vi "Patch data preview core.vi"(6 "Global cycle number among all trials":i32, 9 "Channel to load":enum16{"Red", "Green"}(ring)) -> (1 "Image ref (montage)":T1, 2 "Array":T1[](array[typedef]), 3 "Next state":T2=enum."Idle")   [LabVIEW 2020]
uses:
  Typedefs/Patch viewer internal cluster.ctl
  <vilib>/vision/Image Controls.llb/IMAQ Image.ctl
  Typedefs/Patch viewer states.ctl
  Typedefs/Read Write Enum.ctl
  User Interface/Visualisation/Timelapse Viewer/Globals/gl_Time series viewer globals.vi
  <vilib>/vision/NI_Vision_Development_Module.lvlib
panel:
  out "Array 2":T1[](array[plugin-control])
  out "Coordinates of montage positions":cluster{"X\n\nY":i32[]}[](array[cluster])
  out "Register cluster":T3
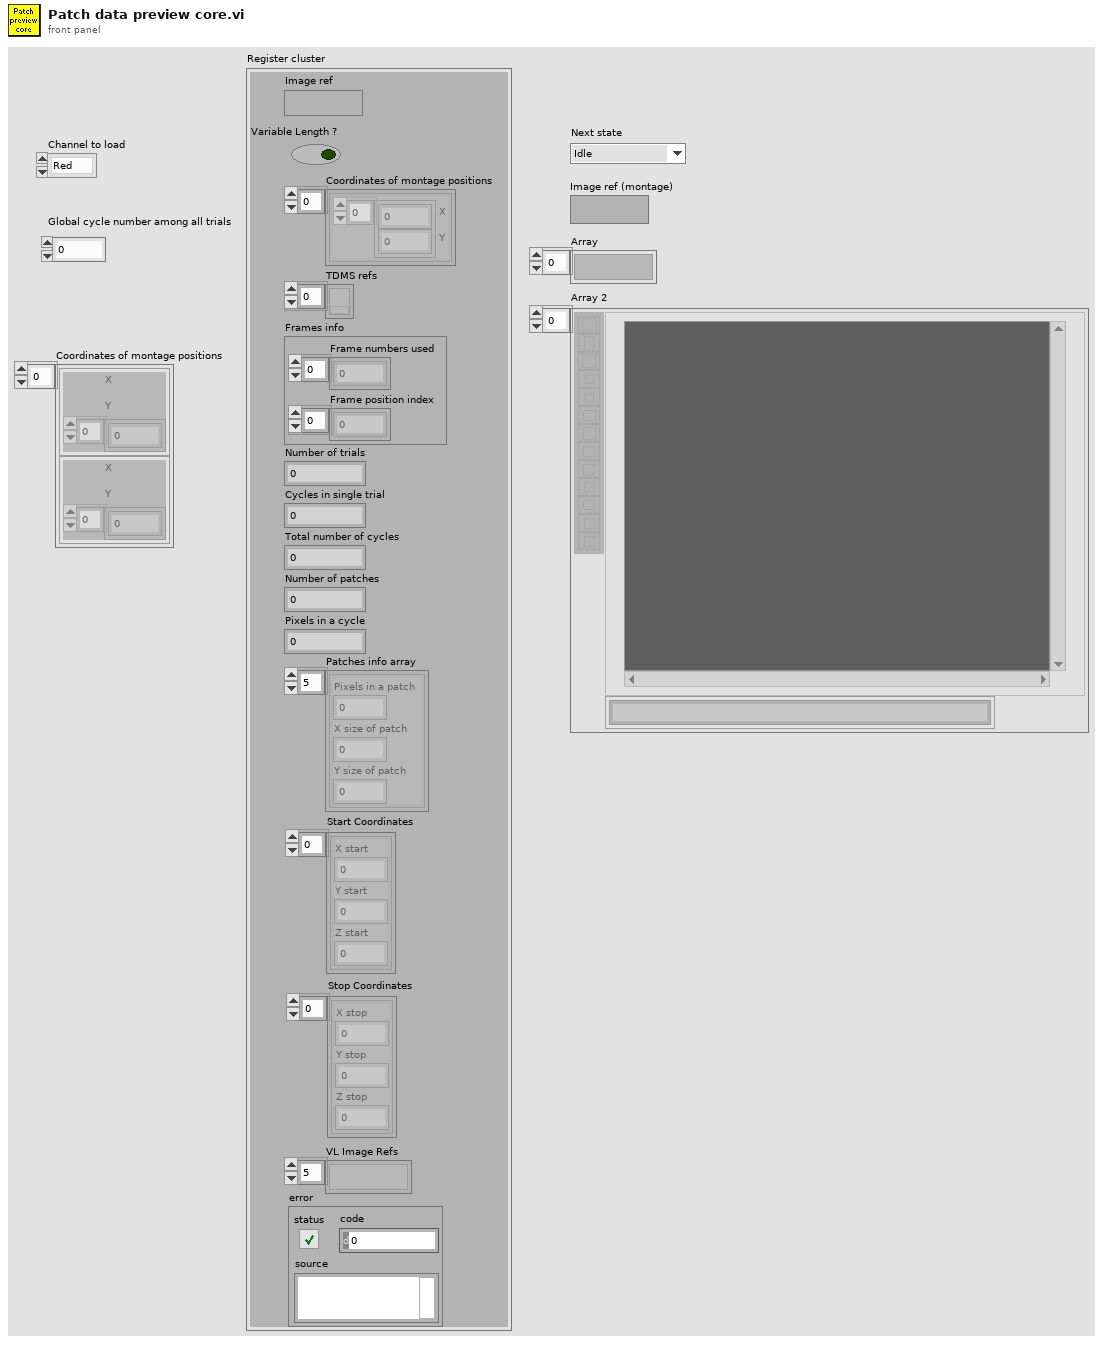
[diagram p1: front panel]
types:
  T1 = typedef "IMAQ Image.ctl" = refnum<image>
  T2 = typedef "Patch viewer states.ctl" = enum16{"Initialise", "Refresh", "Idle", "Error"}
  T3 = typedef "Patch viewer internal cluster.ctl" = cluster{"Image ref":T1, "Variable Length ?":bool, "Coordinates of montage positions":cluster{"X\n\nY":i32[]}[], "TDMS refs":refnum<k34>[], "Frames info":cluster{"Frame numbers used":i32[], "Frame position index":i32[]}, "Number of trials":i32, "Cycles in single trial":i32, "Total number of cycles":i32, "Number of patches":i32, "Pixels in a cycle":i32, "Patches info array":cluster{"Pixels in a patch":i32, "X size of patch":i32, "Y size of patch":i32}[], "Start Coordinates":cluster{"X start":i32, "Y start":i32, "Z start":i32}[], "Stop Coordinates":cluster{"X stop":i32, "Y stop":i32, "Z stop":i32}[], "VL Image Refs":T1[], "error":errorcluster}
  T4 = typedef "Read Write Enum.ctl" = enum16{"Read", "Write"}
  T5 = typedef "Image Type" = u32
  T6 = cluster{"Frame numbers used":i32[], "Frame position index":i32[]}
  T7 = cluster{"Pixels in a patch":i32, "X size of patch":i32, "Y size of patch":i32}[]
  T8 = typedef "Time series viewer refs.ctl" = cluster{"This VI":refnum<vi>, "Image control":refnum<vi>, "AVI Mode ind":refnum<vi>, "Play":refnum<vi>, "Stop":refnum<vi>, "Back":refnum<vi>, "Scrollbar":refnum<vi>, "Video length info":refnum<vi>, "Expected speed values":refnum<vi>, "Intensity":refnum<vi>, "Path":refnum<vi>, "Selection sliders":refnum<vi>, "Speed Graph ref":refnum<vi>, "Frame rate set (fps)":refnum<vi>, "Number of rows to generate":refnum<vi>, "VL Image Array":refnum<vi>, "Image Scrollbar":refnum<vi>, "Channel to load":refnum<vi>, "Colour":refnum<vi>}
  T9 = cluster{"X start":i32, "Y start":i32, "Z start":i32}[]
  T10 = cluster{"X stop":i32, "Y stop":i32, "Z stop":i32}[]
  T11 = typedef "Channel to load.ctl" = enum16{"Show red channel", "Show green channel", "Show both channels"}
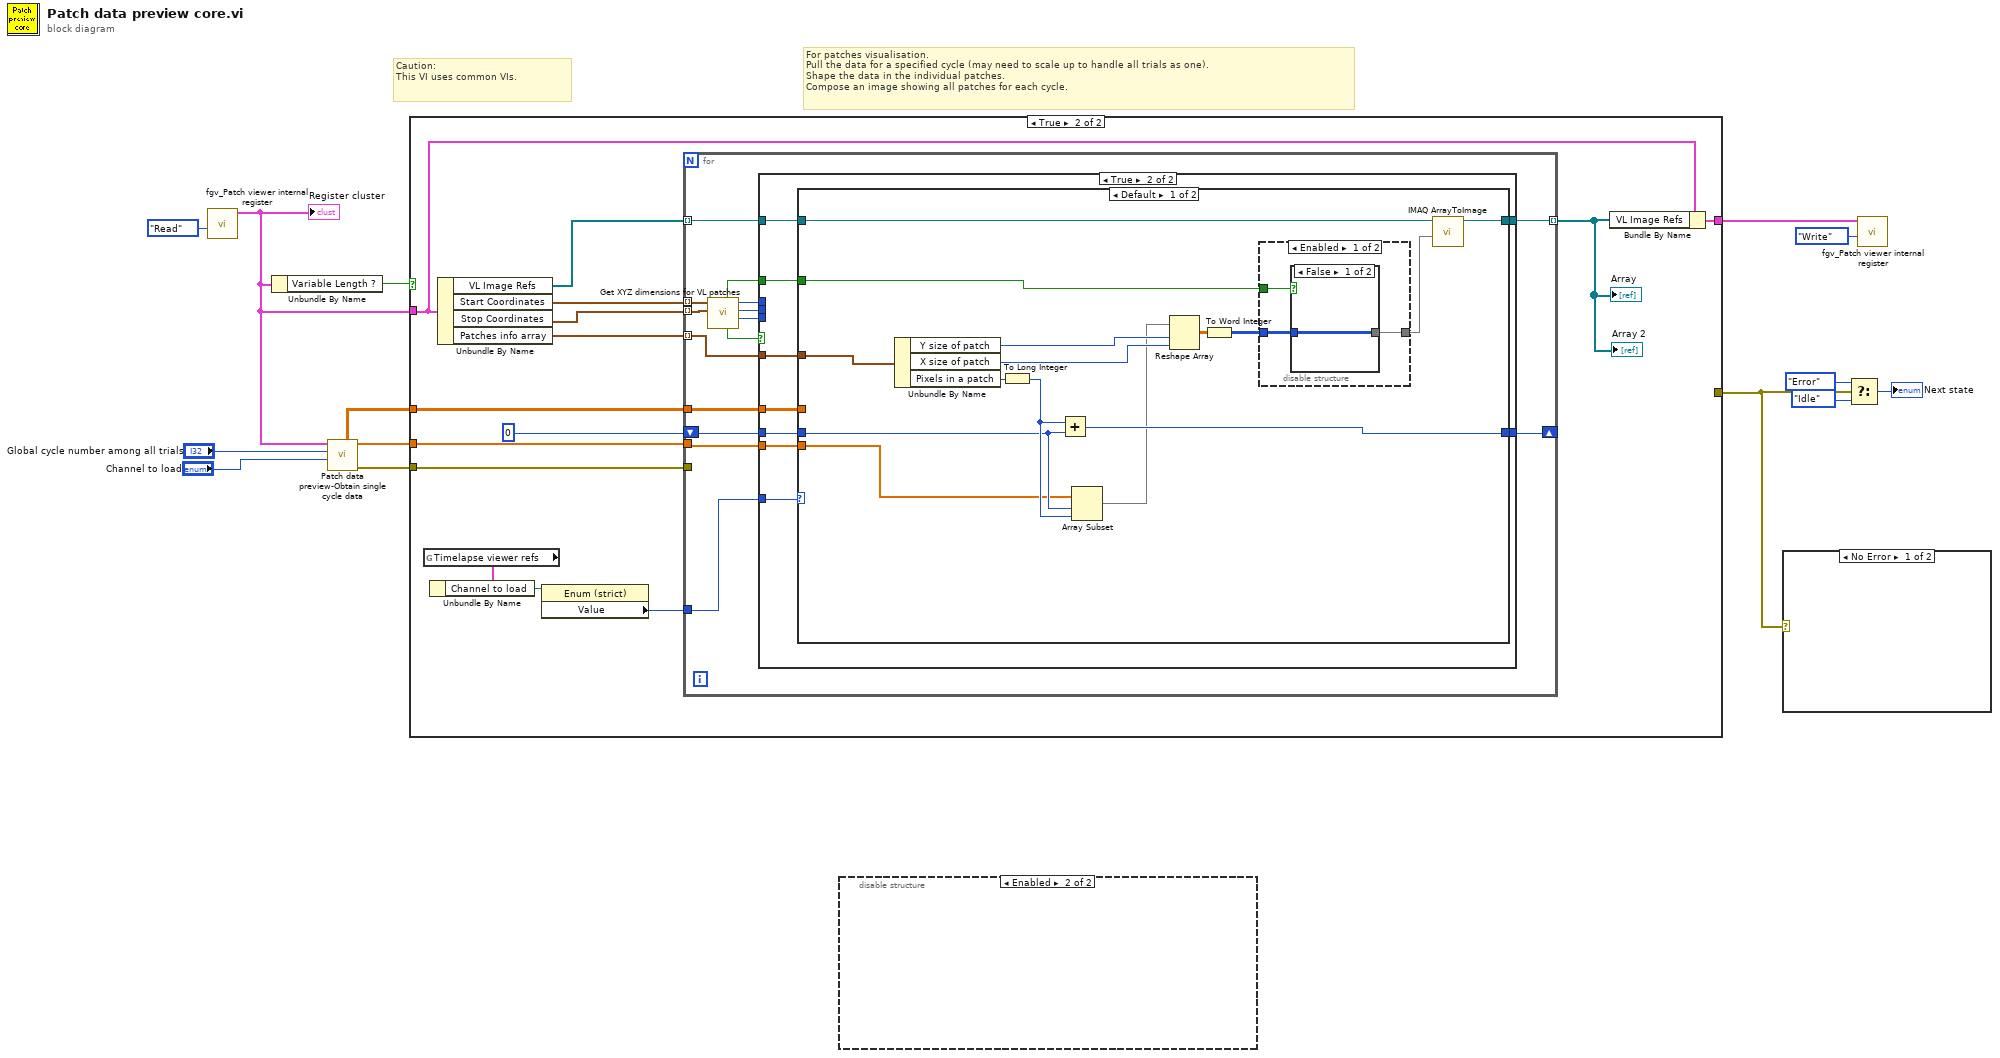
[diagram p0: block diagram]
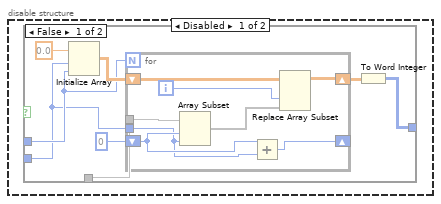
[diagram p2: hidden frame]
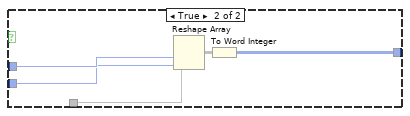
[diagram p3: hidden frame]
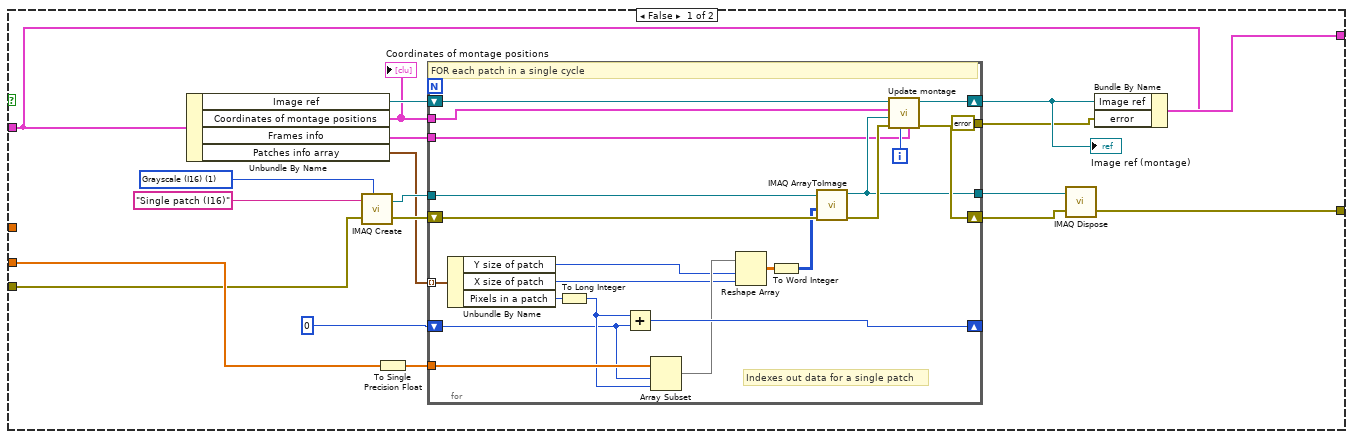
[diagram p4: hidden frame]
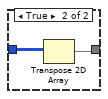
[diagram p6: hidden frame]
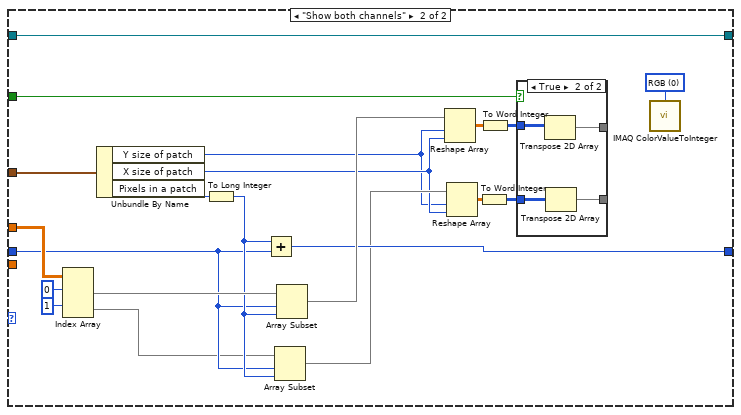
[diagram p8: hidden frame]
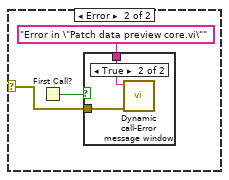
[diagram p10: hidden frame]
diagram:
  # "Caution:\nThis VI uses common VIs."
  # "For patches visualisation.\nPull the data for a specified cycle (may need to scale up to handle all trials as one).\nShape the data in the individual patches.\nCompose an image showing all patches for each cycle."
  n1 = call "fgv_Patch viewer internal register.vi"("Function"=Read_Write_Enum."Read") -> ("Registered setup"=w3:T3)  [unwired: 10 in]
  "Register cluster" <- w3
  n2 = Unbundle By Name(w3) -> ("Variable Length ?"=w1:bool)
  n3 = call "Patch data preview-Obtain single cycle data.vi"("Channel to load"="Channel to load", "Global cycle number among all trials"="Global cycle number among all trials", "Register cluster"=w3) -> ("error out"=w13:errorcluster, "Data from single channel single cycle"=w14:dbl[], "Double channel data"=w2:dbl[][])  [unwired: 6 in]
  n4 = case shown="True" w1 {
    tunnel: w14 -> [w27 w66]
    tunnel: w13 -> [w24 w65]
    tunnel: [w19 w61] -> w5
    tunnel: [w18 _] -> w4
    tunnel: w3 -> [w16 w62]
    tunnel: w2 -> [_ w56]
    frame False {
      w32 = T5 1 items=["Grayscale (U8)", "Grayscale (I16)", "Grayscale (SGL)", "Complex (CSG)", "RGB (U32)", "HSL (U32)", "RGB (U64)", "Grayscale (U16)"] ("Image Type")
      n5 = Unbundle By Name(w16) -> ("Image ref"=w23:T1, "Coordinates of montage positions"=w22:cluster{"X\n\nY":i32[]}[], "Frames info"=w21:T6, "Patches info array"=w20:T7)
      "Coordinates of montage positions" <- w22
      n6 = call "IMAQ Create"("Image Name"="Single patch (I16)", "Image Type"=w32, "error in (no error)"=w24) -> ("New Image"=w30:T1, "error out"=w28:errorcluster)  [unwired: 1 in, 1 out]
      n7 = To Single Precision Float(number=w27) -> (single precision float=w29:sgl[])
      n8 = for {
        tunnel: w20 -> [w55] mode=indexing
        shift-right: [w52] -> _
        shift-left: 0 -> [w37]
        tunnel: w29 -> [w53]
        tunnel: w30 -> [w47]
        tunnel: [w40] -> w26
        shift-right: [w42] -> w25
        shift-left: w28 -> [w46]
        shift-right: [w38] -> w17
        shift-left: w23 -> [w44]
        tunnel: w22 -> [w45]
        tunnel: w21 -> [w39]
        tunnel: [errorcluster {"status"=FALSE, "code"=0, "source"=""} ("error")] -> w15
        i -> [w41]
        # "Indexes out data for a single patch"
        # "FOR each patch in a single cycle"
        n9 = Unbundle By Name(w55) -> ("Y size of patch"=w49:i32, "X size of patch"=w48:i32, "Pixels in a patch"=w54:i32)
        n10 = To Long Integer(number=w54) -> (32bit integer=w51:i32)
        n11 = Add(x=w51, y=w37) -> (x+y=w52:i32)
        n12 = Array Subset "Array Subset"(array=w53, index=w37, length=w51) -> (w50:sgl[])
        n13 = Reshape Array(w50, w49, w48) -> (w35:sgl[][])
        n14 = To Word Integer(number=w35) -> (16bit integer=w36:i16[][])
        n15 = call "IMAQ ArrayToImage"("error in (no error)"=w46, "Image Pixels (I16)"=w36, "Image"=w47) -> ("error out"=w43:errorcluster, "Image Out"=w40:T1)  [unwired: 7 in]
        n16 = call "Update montage.vi"("Frames info"=w39, "Frame's rel. index"=w41, "Error in"=w43, "Single patch image"=w40, "Coordinates of montage positions"=w45, "Image (Montage)"=w44) -> ("error out"=w42:errorcluster, "Image (Montage)"=w38:T1)  [unwired: 4 in]
      }
      "Image ref (montage)" <- w17
      n17 = call "IMAQ Dispose"("Image"=w26, "error in (no error)"=w25) -> ("error out"=w18:errorcluster)  [unwired: 4 in]
      n18 = Bundle By Name(cluster=w16, "Image ref"=w17, "error"=w15) -> (w19:T3)
    }
    frame True {
      n19 = global read "gl_Time series viewer globals.vi" "Timelapse viewer refs"() -> (w59:T8)
      n20 = Unbundle By Name(w59) -> ("Channel to load"=w58:refnum<vi>)
      n21 = Unbundle By Name(w62) -> ("VL Image Refs"=w69:T1[], "Start Coordinates"=w68:T9, "Stop Coordinates"=w67:T10, "Patches info array"=w64:T7)
      n22 = property class="Enum (strict)"(reference=w58) -> ("Value"=w57:T11)  [unwired: 1 in, 2 out]
      n23 = for {
        tunnel: w69 -> [w73] mode=indexing
        tunnel: w68 -> [w84] mode=indexing
        tunnel: w67 -> [w83] mode=indexing
        tunnel: w66 -> [w74]
        tunnel: w65 -> [_]
        tunnel: w64 -> [w77] mode=indexing
        shift-right: [w75] -> _
        shift-left: 0 -> [w76]
        tunnel: [w72] -> w60 mode=indexing
        tunnel: w57 -> [w71]
        tunnel: w56 -> [w70]
        n24 = call "Get XYZ dimensions for VL patches.vi"("Stop coordinates"=w83, "Start coordinates"=w84) -> ("DeltaZ"=w79:i32, "DeltaY"=w80:i32, "DeltaX"=w81:i32, "Single Plane ROI"=w82:bool, "X < Y?"=w78:bool)  [unwired: 4 in, 1 out]
        n25 = case shown="True" w82 {
          tunnel: w81 -> [_ _]
          tunnel: w80 -> [_ _]
          tunnel: w79 -> [_ _]
          tunnel: w78 -> [_ w89]
          tunnel: w77 -> [_ w95]
          tunnel: w76 -> [w85 w94]
          tunnel: [w85 w93] -> w75
          tunnel: w74 -> [_ w92]
          tunnel: w73 -> [w86 w91]
          tunnel: [w86 w90] -> w72
          tunnel: w71 -> [_ w88]
          tunnel: w70 -> [_ w87]
          frame False {
          }
          frame True {
            n26 = case shown="Default" w88 {
              tunnel: w95 -> [w108 w135]
              tunnel: w94 -> [w107 w126]
              tunnel: [w106 w134] -> w93
              tunnel: w92 -> [w105 _]
              tunnel: w91 -> [w104 w118]
              tunnel: [w103 w118] -> w90
              tunnel: w89 -> [w98 w133]
              tunnel: w87 -> [_ w131]
              frame Default {
                n27 = Unbundle By Name(w108) -> ("Y size of patch"=w102:i32, "X size of patch"=w101:i32, "Pixels in a patch"=w110:i32)
                n28 = To Long Integer(number=w110) -> (32bit integer=w109:i32)
                n29 = Add(x=w109, y=w107) -> (x+y=w106:i32)
                n30 = Array Subset "Array Subset"(array=w105, index=w107, length=w109) -> (w100:dbl[])
                n31 = Reshape Array(w100, w102, w101) -> (w99:dbl[][])
                n32 = To Word Integer(number=w99) -> (16bit integer=w97:i16[][])
                n33 = disable-structure shown="Enabled" {
                  disable-tunnel: w98 -> [w113 _]
                  disable-tunnel: w97 -> [w112 w117]
                  disable-tunnel: [w111 w117] -> w96
                  frame Enabled {
                    n34 = case shown="False" w113 {
                      tunnel: w112 -> [w114 w116]
                      tunnel: [w114 w115] -> w111
                      frame False {
                      }
                      frame True {
                        n35 = Transpose 2D Array(2D array=w116) -> (transposed array=w115:i16[][])
                      }
                    }
                  }
                  frame Disabled {
                  }
                }
                n36 = call "IMAQ ArrayToImage"("Image Pixels (I16)"=w96, "Image"=w104) -> ("Image Out"=w103:T1)  [unwired: 8 in, 1 out]
              }
              frame "Show both channels" {
                w119 = u16 0 items=["RGB", "HSL", "HSV", "HSI"] ("Color Mode")
                n37 = Index Array(array=w131, index (row) #1=0 ("index (row)"), index (row) #2=1 ("index (row)")) -> (element #1=w128:dbl[], element #2=w125:dbl[])  [unwired: 2 in]
                n38 = Unbundle By Name(w135) -> ("Y size of patch"=w122:i32, "X size of patch"=w123:i32, "Pixels in a patch"=w138:i32)
                n39 = To Long Integer(number=w138) -> (32bit integer=w127:i32)
                n40 = Add(x=w127, y=w126) -> (x+y=w134:i32)
                n41 = Array Subset "Array Subset"(array=w125, index=w126, length=w127) -> (w124:dbl[])
                n42 = Array Subset "Array Subset"(array=w128, index=w126, length=w127) -> (w137:dbl[])
                n43 = Reshape Array(w137, w122, w123) -> (w136:dbl[][])
                n44 = Reshape Array(w124, w122, w123) -> (w121:dbl[][])
                n45 = To Word Integer(number=w121) -> (16bit integer=w120:i16[][])
                n46 = To Word Integer(number=w136) -> (16bit integer=w132:i16[][])
                n47 = case shown="True" w133 {
                  tunnel: w132 -> [w140 w144]
                  tunnel: [w140 w143] -> _
                  tunnel: w120 -> [w139 w142]
                  tunnel: [w139 w141] -> _
                  frame False {
                  }
                  frame True {
                    n48 = Transpose 2D Array(2D array=w144) -> (transposed array=w143:i16[][])
                    n49 = Transpose 2D Array(2D array=w142) -> (transposed array=w141:i16[][])
                  }
                }
                n50 = call "IMAQ ColorValueToInteger"("Color Mode"=w119) -> ()  [unwired: 4 in, 4 out]
              }
            }
          }
        }
      }
      "Array" <- w60
      "Array 2" <- w60
      n51 = Bundle By Name(cluster=w62, "VL Image Refs"=w60) -> (w61:T3)
    }
  }
  n52 = disable-structure shown="Enabled" {
    frame Disabled {
      n53 = case shown="False" {
        selector: _ -> [_ _]
        tunnel: _ -> [w146 w163]
        tunnel: _ -> [w145 w162]
        tunnel: _ -> [w151 w164]
        tunnel: [w147 w161] -> _
        frame False {
          n54 = Initialize Array(0.0, w145, w146) -> (w150:dbl[][])
          n55 = for {
            N: w146 -> [_]
            tunnel: w151 -> [w157]
            shift-right: [w159] -> w148
            shift-left: w150 -> [w160]
            shift-right: [w154] -> _
            shift-left: 0 -> [w156]
            tunnel: w145 -> [w155]
            i -> [w158]
            n56 = Array Subset(array=w157, index=w156, length=w155) -> (w153:void[])
            n57 = Add(x=w156, y=w155) -> (x+y=w154:i32)
            n58 = Replace Array Subset(array=w160, new element=w153, index (col)=w158) -> (w159:dbl[][])  [unwired: 1 in]
          }
          n59 = To Word Integer(number=w148) -> (16bit integer=w147:i16[][])
        }
        frame True {
          n60 = Reshape Array(w164, w163, w162) -> (w165:void[][])
          n61 = To Word Integer(number=w165) -> (16bit integer=w161:i16[][])
        }
      }
    }
    frame Enabled {
    }
  }
  n62 = case shown="No Error" w4 {
    selector: w4 -> [_ w167]
    frame No Error {
    }
    frame Error {
      n63 = First Call?() -> (First Call?: T/F=w168:bool)
      n64 = case shown="True" w168 {
        tunnel: w167 -> [_ w170]
        tunnel: "Error in \"Patch data preview core.vi\"" ("Error Message") -> [_ w169]
        frame False {
        }
        frame True {
          n65 = call "Dynamic call-Error message window.vi"("error in (no error)"=w170, "Error Message"=w169) -> ()  [unwired: 9 in, 1 out]
        }
      }
    }
  }
  n66 = Select(t=Patch_viewer_states."Error" ("States"), s=w4, f=Patch_viewer_states."Idle" ("States")) -> (s? t:f=→"Next state":T2)
  n67 = call "fgv_Patch viewer internal register.vi"("Function"=Read_Write_Enum."Write", "Registered setup"=w5) -> ()  [unwired: 9 in, 1 out]
